vi "Select Records.vi"(8 "Error In (no error)":errorcluster, 11 "Database Interactions In":refnum<class "Database Interactions.lvclass">) -> (0 "Error Out":errorcluster, 3 "Database Interactions Out":refnum<class "Database Interactions.lvclass">)   [LabVIEW 2023, in "Database Interactions.lvclass"]
uses:
  Database Interactions.lvclass
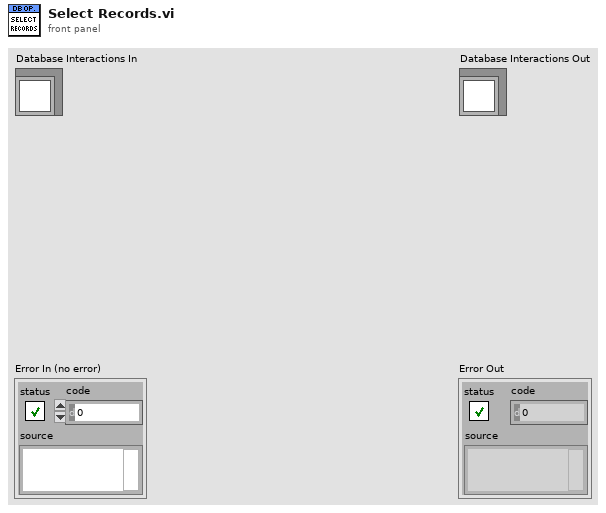
[diagram p1: front panel]
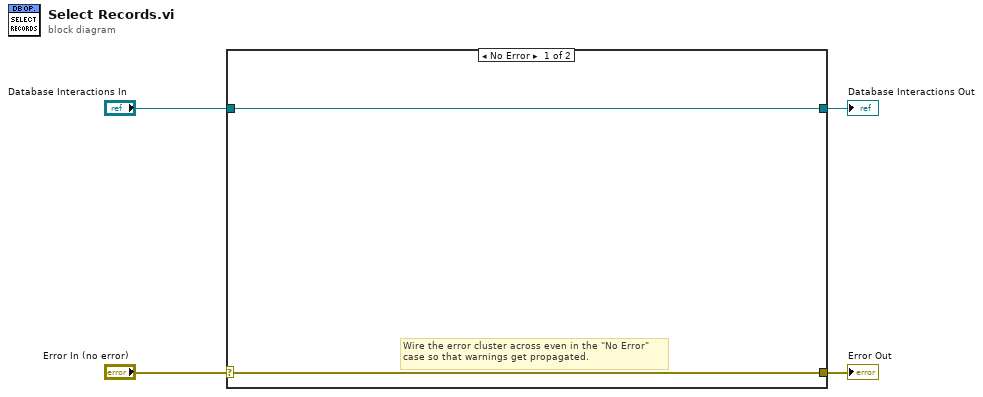
[diagram p0: block diagram]
diagram:
  n1 = case shown="No Error" "Error In (no error)" {
    selector: "Error In (no error)" -> [w5 w8]
    tunnel: [w5 w8] -> w3
    tunnel: [w6 w7] -> w1
    tunnel: "Database Interactions In" -> [w6 w7]
    frame No Error {
      # "Wire the error cluster across even in the \"No Error\"\ncase so that warnings get propagated."
    }
    frame Error {
    }
  }
  "Error Out" <- w3
  "Database Interactions Out" <- w1
